vi "XML-String in Namen-Array.vi"(1 "XML-String":string) -> (0 "Namen (ohne Cluster)":string[](array[string]))   [LabVIEW 2020, in "Anlagenuebersicht.lvlib" / "VisBx Anzeige.lvlib"]
uses:
  VisBx Anzeige.lvlib
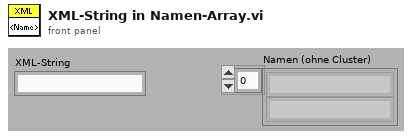
[diagram p1: front panel]
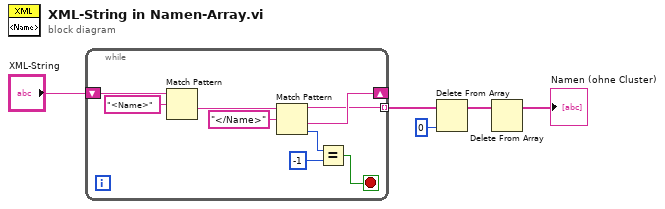
[diagram p0: block diagram]
diagram:
  n1 = while {
    shift-right: [w10] -> _
    shift-left: "XML-String" -> [w12]
    tunnel: [w9] -> w4 mode=indexing
    stop <- w6 stop-if-true
    n2 = Match Pattern(string=w12, regular expression="<Name>") -> (after substring=w11:string)  [unwired: 4 out]
    n3 = Match Pattern(string=w11, regular expression="</Name>") -> (before substring=w9:string, after substring=w10:string, offset past match=w8:i32)  [unwired: 2 out]
    n4 = Equal?(x=w8, y=-1) -> (x = y?=w6:bool)
  }
  n5 = Delete From Array(array=w4, index=0 ("Index")) -> (array with subset deleted=w2:string[])  [unwired: 1 in, 1 out]
  n6 = Delete From Array(array=w2) -> (array with subset deleted=→"Namen (ohne Cluster)":string[])  [unwired: 2 in, 1 out]
